vi "PDF Report Facade.vi"(0 "Data In":T4={"Document"=refnum, "Writer"=refnum, "Default Font"=refnum, "Default Font cluster"={"Name"="Helvetica", "Size"=12.0, "Color"=0, "Style"={"Bold"=FALSE, "Italic"=FALSE, "Underline"=FALSE, "Strikeout"=FALSE}}, "Path"=path "", "Unit (default = mm)"=enum."mm", "Paragraphe cluster"={" Aligment"=enum."Select", "Line spacing"=enum."Select"}, "Pages dimensions [ ]"=[], "Captions"={"Image"={"Caption"="", "Separator"="", "Position"=enum."Above"}, "Image counter"=0, "Table"={"Caption"="", "Separator"="", "Position"=enum."Above"}, "Table counter"=0, "Font"={"Name"="", "Size"=-1.0, "Color"=0, "Style"={"Bold"=FALSE, "Italic"=FALSE, "Underline"=FALSE, "Strikeout"=FALSE}}}, "Header"=[], "Footer"=[], "Watermark "={"Show? (F)"=FALSE, "Type"=enum."Text", "Opacity (%)"=10.0, "Rotate(°)"=0.0, "Position"={"Position"=enum."Center (text section)", "X"=0.0, "Y"=0.0}, "Image path"=path "", "Scaled(%)"=100.0, "Image refnum"=refnum, "Text"="CONFIDENTIAL", "Font"={"Name"="", "Size"=-1.0, "Color"=0}, "Font refnum"=refnum, "Alignment"=enum."Center", "Automatic"=FALSE}, "Actual VI name"="", "System Fonts"={"Font name [ ]"=[], "Font and file names [ ]"=[]}}, 2 "Display State In":T2, 3 "Container State":T3) -> (6 "Data Out":T4={"Document"=refnum, "Writer"=refnum, "Default Font"=refnum, "Default Font cluster"={"Name"="Helvetica", "Size"=12.0, "Color"=0, "Style"={"Bold"=FALSE, "Italic"=FALSE, "Underline"=FALSE, "Strikeout"=FALSE}}, "Path"=path "", "Unit (default = mm)"=enum."mm", "Paragraphe cluster"={" Aligment"=enum."Select", "Line spacing"=enum."Select"}, "Pages dimensions [ ]"=[], "Captions"={"Image"={"Caption"="", "Separator"="", "Position"=enum."Above"}, "Image counter"=0, "Table"={"Caption"="", "Separator"="", "Position"=enum."Above"}, "Table counter"=0, "Font"={"Name"="", "Size"=-1.0, "Color"=0, "Style"={"Bold"=FALSE, "Italic"=FALSE, "Underline"=FALSE, "Strikeout"=FALSE}}}, "Header"=[], "Footer"=[], "Watermark "={"Show? (F)"=FALSE, "Type"=enum."Text", "Opacity (%)"=10.0, "Rotate(°)"=0.0, "Position"={"Position"=enum."Center (text section)", "X"=0.0, "Y"=0.0}, "Image path"=path "", "Scaled(%)"=100.0, "Image refnum"=refnum, "Text"="CONFIDENTIAL", "Font"={"Name"="", "Size"=-1.0, "Color"=0}, "Font refnum"=refnum, "Alignment"=enum."Center", "Automatic"=FALSE}, "Actual VI name"="", "System Fonts"={"Font name [ ]"=[], "Font and file names [ ]"=[]}}, 7 "Display State Out":T2, 8 "Action":T1)   [LabVIEW 2012, in "PDF Report.xctl"]
uses:
  PDF Report.xctl
  PDF Report Data.ctl
  C:/Users/MaxCorp/Documents/TopPerm - Base/DLL/itextsharp.dll
  DLL/itextsharp.dll
  Font cluster.ctl
  Font size.ctl
  Font color.ctl
  Unit.ctl
  Paragraphe cluster.ctl
  Texte alignement.ctl
  Line spacing.ctl
  Page dimensions.ctl
  Page Orientation.ctl
  Image or Table Caption.ctl
  Header Footer [ ].ctl
  Header Footer cluster.ctl
  Header Footer Type.ctl
  Header footer horiz alignment.ctl
  Cell Vertical alignment.ctl
  Page number.ctl
  Header Footer Line.ctl
  Watermark cluster2.ctl
  Watermark Position.ctl
  System Fonts.ctl
  <vilib>/_xctls/Container State.ctl
  PDF Report State.ctl
  <vilib>/_xctls/Action.ctl
  <vilib>/Utility/miscctls.llb/LVPointTypeDef.ctl
  <vilib>/_xctls/XControlSupport.lvlib
panel:
  in  "String":string="  \nPDF"
  # "X"
  # "Y"
  # "X"
  # "Y"
  # "X"
  # "Y"
  # "X"
  # "Y"
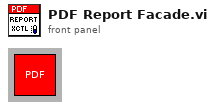
[diagram p1: front panel]
types:
  T1 = typedef "XControlSupport.lvlib/Action.ctl" = cluster{"Data Changed?":bool, "State Changed?":bool, "Action Name":string}
  T2 = typedef "PDF Report.xctl/PDF Report State.ctl" = cluster{"Action":string, "Clear":bool}
  T3 = typedef "XControlSupport.lvlib/Container State.ctl" = cluster{"Indicator?":bool, "Run Mode?":bool, " Refnum":refnum<vi>}
  T4 = typedef "PDF Report.xctl/PDF Report Data.ctl" = cluster{"Document":refnum<k24>, "Writer":refnum<k24>, "Default Font":refnum<k24>, "Default Font cluster":T5, "Path":path, "Unit (default = mm)":T8, "Paragraphe cluster":T9, "Pages dimensions [ ]":T12[], "Captions":cluster{"Image":T14, "Image counter":u16, "Table":T14, "Table counter":u16, "Font":T5}, "Header":T15, "Footer":T15, "Watermark ":T22, "Actual VI name":string, "System Fonts":T24}
  T5 = typedef "Font cluster.ctl" = cluster{"Name":string, "Size":T6, "Color":T7, "Style":cluster{"Bold":bool, "Italic":bool, "Underline":bool, "Strikeout":bool}}
  T6 = typedef "Font size.ctl" = sgl
  T7 = typedef "Font color.ctl" = u32
  T8 = typedef "Unit.ctl" = enum16{"inch", "mm"}
  T9 = typedef "Paragraphe cluster.ctl" = cluster{" Aligment":T10, "Line spacing":T11}
  T10 = typedef "Texte alignement.ctl" = enum16{"Select", "CENTER", "JUSTIFY", "LEFT", "RIGHT"}
  T11 = typedef "Line spacing.ctl" = enum16{"Select", "1.0", "1.5", "2.0"}
  T12 = typedef "Page dimensions.ctl" = cluster{"Start at page":i32, "Orientation":T13, "widht":sgl, "height":sgl, "Margin left":sgl, "Margin right":sgl, "Margin top":sgl, "Margin bottom":sgl}
  T13 = typedef "Page Orientation.ctl" = enum16{"Portrait", "Landscape"}
  T14 = typedef "Image or Table Caption.ctl" = cluster{"Caption":string, "Separator":string, "Position":enum16{"Above", "Below"}}
  T15 = typedef "Header Footer [ ].ctl" = T16[]
  T16 = typedef "Header Footer cluster.ctl" = cluster{"Start page":i32, "Type":T17, "Alignment":T18, "Vertical Alignement":T19, "Image (%)":sgl, "Page #":T20, "Text":string, "Path":string, "Font":T5, "Font refnum":refnum<k24>, "Line":cluster{"Line":T21, "Thickness (points)":sgl, "Colour":T7}}
  T17 = typedef "Header Footer Type.ctl" = enum16{"Select", "Text", "Text + hyperlink", "Page number", "Image", "Image + hyperlink"}
  T18 = typedef "Header footer horiz alignment.ctl" = enum16{"Left", "Center", "Right"}
  T19 = typedef "Cell Vertical alignment.ctl" = enum16{"TOP", "MIDDLE", "BOTTOM"}
  T20 = typedef "Page number.ctl" = cluster{"Text 1":string, "Text 2":string, "Text 3":string}
  T21 = typedef "Header Footer Line.ctl" = enum16{"No line", "Horizontal line"}
  T22 = typedef "Watermark cluster2.ctl" = cluster{"Show? (F)":bool, "Type":enum16{"Image", "Text"}, "Opacity (%)":sgl, "Rotate(°)":sgl, "Position":cluster{"Position":T23, "X":sgl, "Y":sgl}, "Image path":path, "Scaled(%)":sgl, "Image refnum":refnum<k24>, "Text":string, "Font":cluster{"Name":string, "Size":T6, "Color":T7}, "Font refnum":refnum<k24>, "Alignment":T18, "Automatic":bool}
  T23 = typedef "Watermark Position.ctl" = enum16{"Absolute", "Center (page)", "Center (text section)"}
  T24 = typedef "System Fonts.ctl" = cluster{"Font name [ ]":string[], "Font and file names [ ]":cluster{"Font name":string, "File name":string}[]}
  T25 = typedef "LVPointTypeDef.ctl" = cluster{"Horizontal":i16, "Vertical":i16}
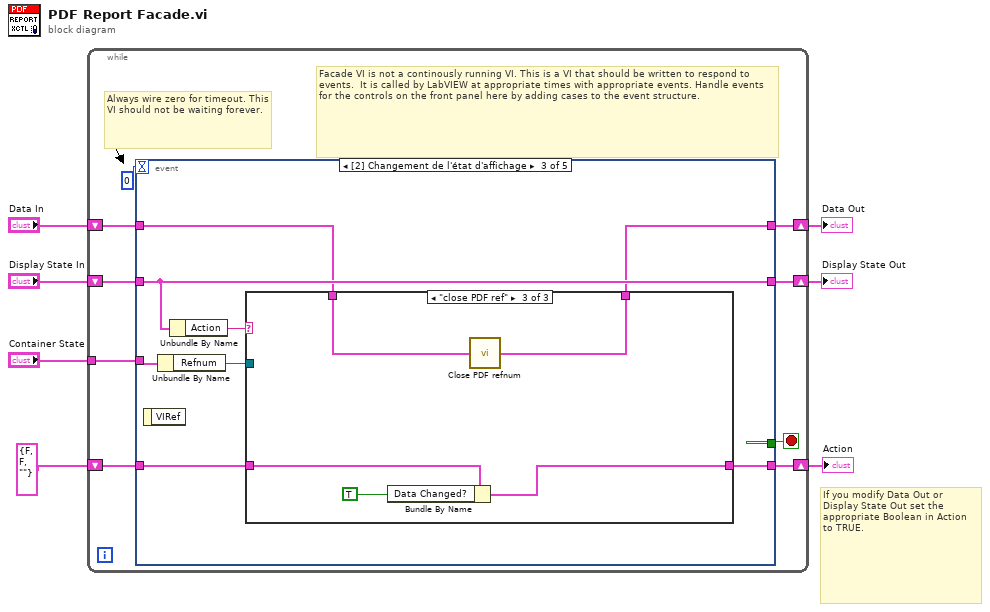
[diagram p0: block diagram]
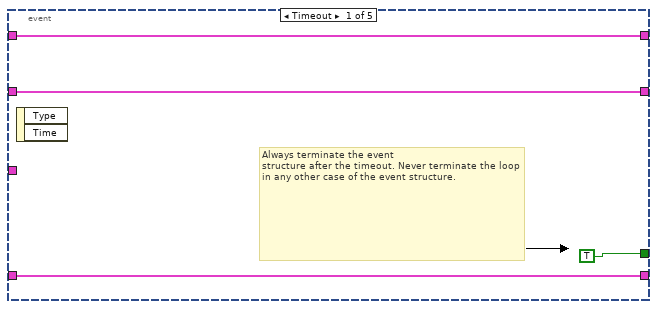
[diagram p2: hidden frame]
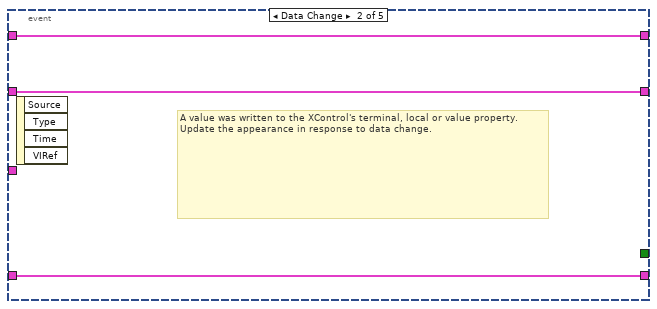
[diagram p3: hidden frame]
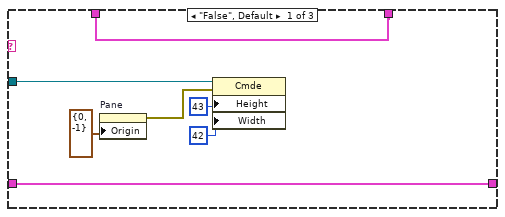
[diagram p4: hidden frame]
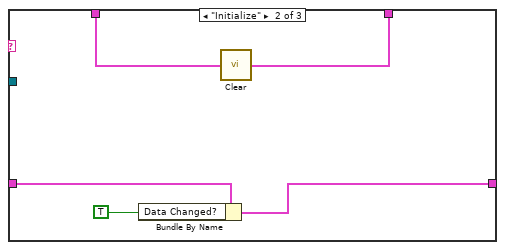
[diagram p5: hidden frame]
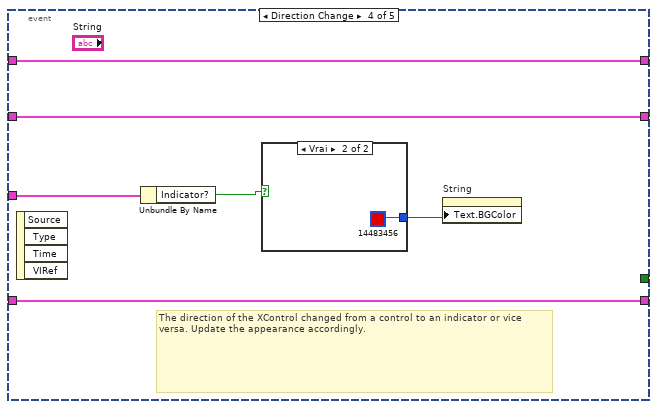
[diagram p6: hidden frame]
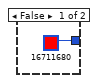
[diagram p7: hidden frame]
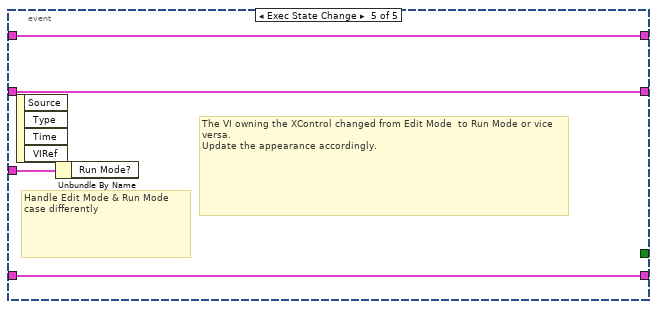
[diagram p8: hidden frame]
diagram:
  # "If you modify Data Out or\nDisplay State Out set the\nappropriate Boolean in Action\nto TRUE."
  n1 = while {
    shift-right: [w15] -> w4
    shift-left: "Display State In" -> [w16]
    tunnel: "Container State" -> [w12]
    shift-right: [w10] -> w7
    shift-left: "Data In" -> [w11]
    shift-right: [w8] -> w2
    shift-left: T1 {"Data Changed?"=FALSE, "State Changed?"=FALSE, "Action Name"=""} ("Action") -> [w9]
    stop <- w14 stop-if-true
    # "Facade VI is not a continously running VI. This is a VI that should be written to respond to events.  It is called by LabVIEW at appropriate times with appropriate events. Handle events for the controls on the front panel here by adding cases to the event structure."
    # "Always wire zero for timeout. This\nVI should not be waiting forever."
    n2 = event shown="[2] Changement de l'état d'affichage" {
      selector: _ -> [_ _ _ _ _]
      dyn-events: _ -> [_ _ _ _ _]
      timeout: 0 -> [_ _ _ _ _]
      tunnel: w16 -> [w18 w22 w30 w53 w59]
      tunnel: [w18 w22 w30 w53 w59] -> w15
      tunnel: [TRUE _ _ _ _] -> w14
      tunnel: w12 -> [_ _ w31 w54 w60]
      tunnel: w11 -> [w17 w23 w25 w52 w58]
      tunnel: [w17 w23 w24 w52 w58] -> w10
      tunnel: [w19 w21 w26 w51 w57] -> w8
      tunnel: w9 -> [w19 w21 w27 w51 w57]
      event Timeout {
        # "Always terminate the event\nstructure after the timeout. Never terminate the loop in any other case of the event structure."
        n3 = event-data() -> ()  [unwired: 3 out]
      }
      event Data Change {
        # "A value was written to the XControl's terminal, local or value property.\nUpdate the appearance in response to data change."
        n4 = event-data() -> ()  [unwired: 5 out]
      }
      event Display State Change {
        n5 = event-data() -> ()  [unwired: 2 out]
        n6 = Unbundle By Name(w31) -> ("Refnum"=w28:refnum<vi>)
        n7 = Unbundle By Name(w30) -> ("Action"=w29:string)
        n8 = case shown="\"close PDF ref\"" w29 {
          tunnel: w28 -> [w37 _ _]
          tunnel: w27 -> [w36 w43 w47]
          tunnel: [w36 w41 w46] -> w26
          tunnel: w25 -> [w35 w40 w44]
          tunnel: [w35 w39 w45] -> w24
          frame "False", Default {
            n9 = property on="Pane" class="Pann"("Origin"=T25 {"Horizontal"=0, "Vertical"=-1}) -> (error out=w34:errorcluster)  [unwired: 2 in, 1 out]
            n10 = property class="Cmde"(reference=w37, error in=w34, "Height"=u32 43 ("XControl:Container Bounds:Height"), "Width"=u32 42 ("XControl:Container Bounds:Height")) -> ()  [unwired: 2 out]
          }
          frame "Initialize" {
            n11 = Bundle By Name(cluster=w43, "Data Changed?"=TRUE) -> (w41:T1)
            n12 = call "Clear.vi"("Data"=w40) -> ("Data OUT"=w39:T4)
          }
          frame "close PDF ref" {
            n13 = Bundle By Name(cluster=w47, "Data Changed?"=TRUE) -> (w46:T1)
            n14 = call "Close PDF refnum.vi"("Data IN"=w44) -> ("Data OUT"=w45:T4)
          }
        }
      }
      event Direction Change {
        # "The direction of the XControl changed from a control to an indicator or vice versa. Update the appearance accordingly."
        n15 = event-data() -> ()  [unwired: 5 out]
        n16 = Unbundle By Name(w54) -> ("Indicator?"=w50:bool)
        n17 = case shown="Vrai" w50 {
          tunnel: [u32 16711680 ("Color Box") u32 14483456 ("Color Box")] -> w49
          frame False {
          }
          frame True {
          }
        }
        n18 = property on="String" class="Ch"("Text.BGColor"=w49) -> ()  [unwired: 2 in, 2 out]
      }
      event Exec State Change {
        # "The VI owning the XControl changed from Edit Mode  to Run Mode or vice versa.\nUpdate the appearance accordingly."
        # "Handle Edit Mode & Run Mode\ncase differently"
        n19 = event-data() -> ()  [unwired: 5 out]
        n20 = Unbundle By Name(w60) -> ()  [unwired: 1 out]
      }
    }
  }
  "Display State Out" <- w4
  "Data Out" <- w7
  "Action" <- w2
